vi "AI init scada.vi"(10 "N_param":i32) -> (0 "error":errorcluster, 3 "AI":T1)   [LabVIEW 2019, in "Inputs.lvlib"]
uses:
  Inputs.lvlib
  Ctl/AI scada.ctl
panel:
  # "Analog parameters"
  # "Description of analog parameters"
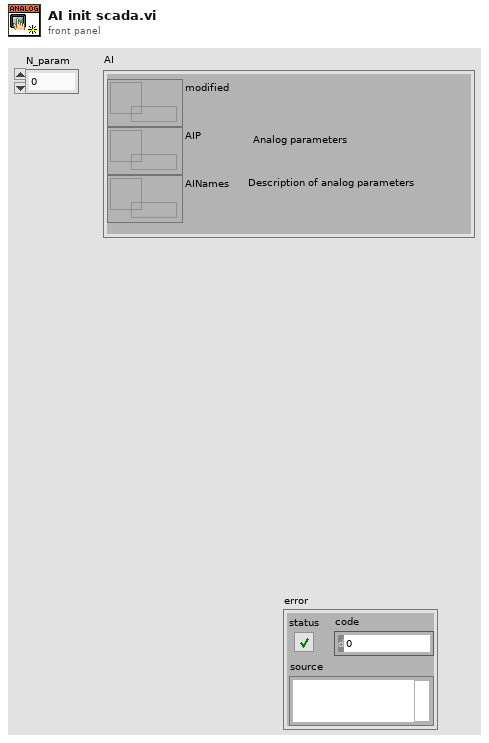
[diagram p1: front panel]
types:
  T1 = typedef "Inputs.lvlib/AI scada.ctl" = cluster{"modified":refnum<data-value>, "AIP":refnum<data-value>, "AINames":refnum<data-value>}
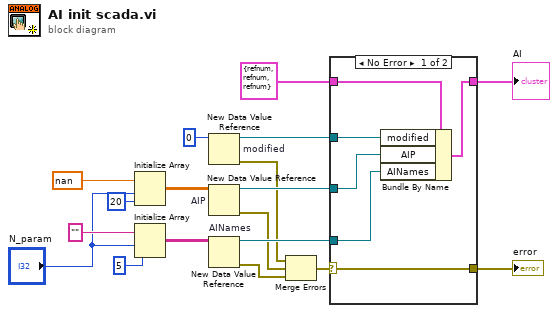
[diagram p0: block diagram]
diagram:
  n1 = Initialize Array(nan ("AIP"), "N_param", 20 ("dimension size")) -> (w7:dbl[][])
  n2 = Initialize Array("" ("AINames"), "N_param", 5 ("dimension size")) -> (w14:string[][])
  n3 = New Data Value Reference "modified"(data value=u8 0 ("modified")) -> (data value reference=w2:refnum<data-value>, error out=w3:errorcluster)  [unwired: 1 in]
  n4 = New Data Value Reference "AIP"(data value=w7) -> (data value reference=w6:refnum<data-value>, error out=w4:errorcluster)  [unwired: 1 in]
  n5 = New Data Value Reference "AINames"(data value=w14) -> (data value reference=w13:refnum<data-value>, error out=w8:errorcluster)  [unwired: 1 in]
  n6 = Merge Errors(w3, w4, w8) -> (w5:errorcluster)
  n7 = case shown="No Error" w5 {
    selector: w5 -> [w22 w26]
    tunnel: w6 -> [w20 _]
    tunnel: w13 -> [w21 _]
    tunnel: [w22 w26] -> w11
    tunnel: T1 {"modified"=refnum, "AIP"=refnum, "AINames"=refnum} ("AI") -> [w24 w25]
    tunnel: [w23 w25] -> w9
    tunnel: w2 -> [w19 _]
    frame No Error {
      n8 = Bundle By Name(cluster=w24, "modified"=w19, "AIP"=w20, "AINames"=w21) -> (w23:T1)
    }
    frame Error {
    }
  }
  "error" <- w11
  "AI" <- w9
